vi "模拟量输入自动测试一组_fast_OK.vi"(8 "AD选择？":bool, 9 "DSP选择？":bool, 11 "第几个":i32) -> ()   [LabVIEW 2010]
uses:
  全局量/试验配置信息.vi
panel:
  in  "AD测试值":dbl[](array[numeric])
  in  "DSP测试值":dbl[](array[numeric])
  # "从0开始"
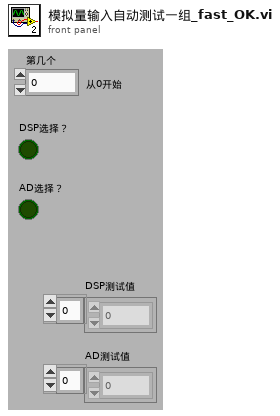
[diagram p1: front panel]
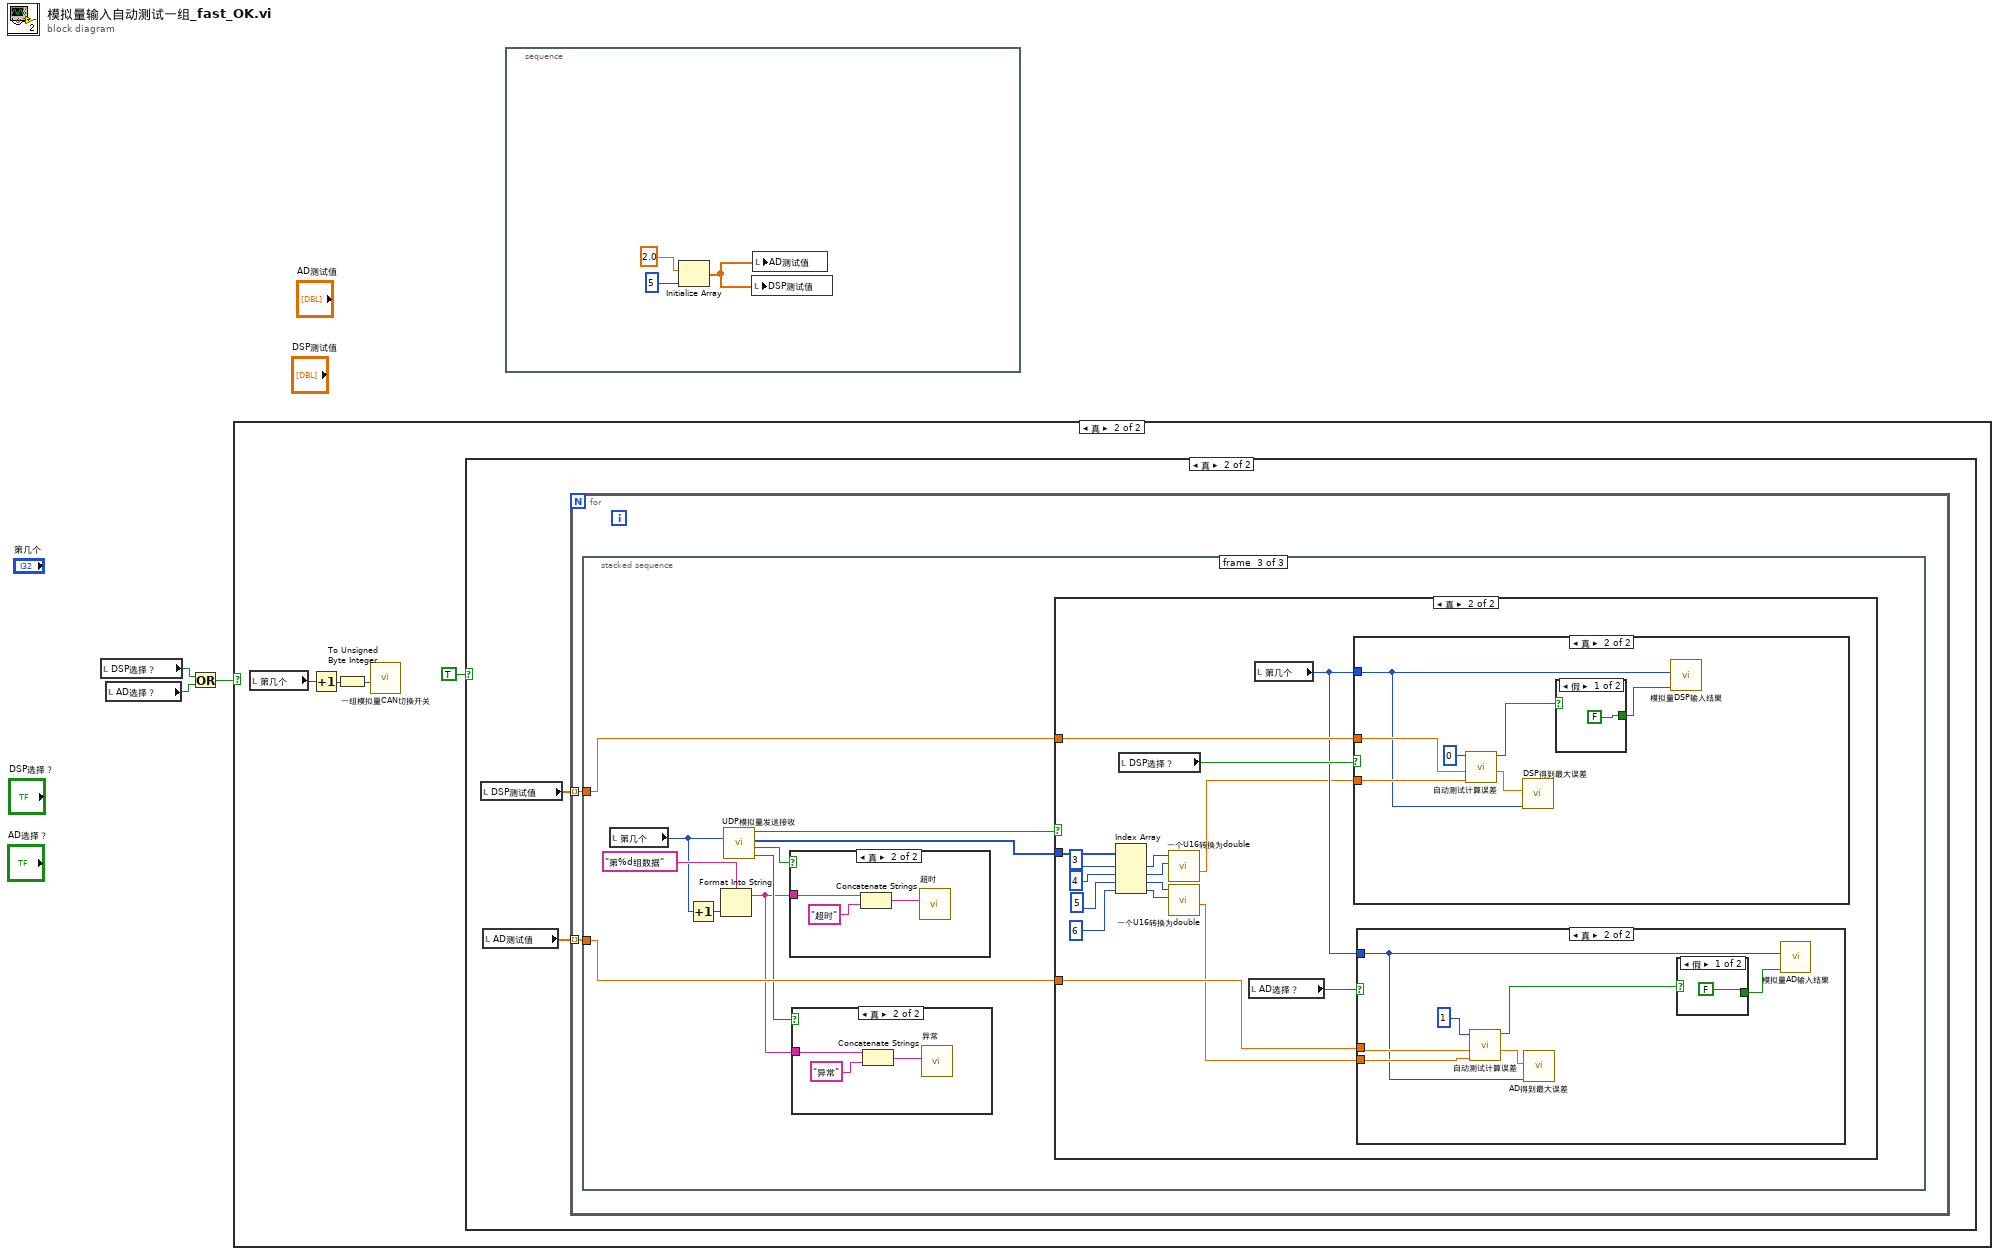
[diagram p0: block diagram]
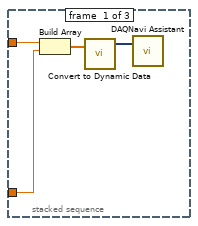
[diagram p4: hidden frame]
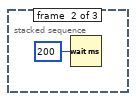
[diagram p5: hidden frame]
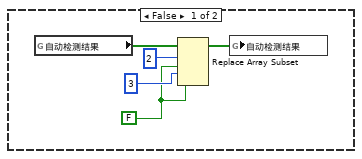
[diagram p8: hidden frame]
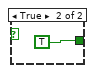
[diagram p10: hidden frame]
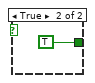
[diagram p12: hidden frame]
diagram:
  n1 = local read "DSP选择？"() -> (w2:bool)
  n2 = local read "AD选择？"() -> (w3:bool)
  n3 = Or(x=w2, y=w3) -> (x .or. y?=w1:bool)
  n4 = case shown="真" w1 {
    frame False {
    }
    frame True {
      n5 = local read "第几个"() -> (w7:i32)
      n6 = Increment(x=w7) -> (x+1=w5:i32)
      n7 = To Unsigned Byte Integer(number=w5) -> (unsigned 8bit integer=w6:u8)
      n8 = call "一组模拟量CAN切换开关.vi"("第几组数据"=w6) -> ()  [unwired: 10 in, 1 out]
      n9 = case shown="真" TRUE {
        frame False {
        }
        frame True {
          n10 = local read "DSP测试值"() -> (w9:dbl[])
          n11 = local read "AD测试值"() -> (w8:dbl[])
          n12 = for {
            tunnel: w9 -> [w11] mode=indexing
            tunnel: w8 -> [w10] mode=indexing
            n13 = stacked-sequence {
              tunnel: w11 -> [w13 _ w26]
              tunnel: w10 -> [w12 _ w25]
              frame #0 {
                n14 = Build Array(w13, w12) -> (w15:dbl[])
                n15 = call "Convert to Dynamic Data"("Array"=w15) -> ("Dynamic Data Type"=w14:dynamicdata)  [unwired: 3 out]
                n16 = call "DAQNavi Assistant"("data in(DDT)"=w14) -> ()  [unwired: 2 in, 17 out]
              }
              frame #1 {
                n17 = Wait (ms)(milliseconds to wait=u32 200 ("等待时间（毫秒）")) -> ()  [unwired: 1 out]
              }
              frame #2 {
                n18 = local read "第几个"() -> (w18:i32)
                n19 = Increment(x=w18) -> (x+1=w19:i32)
                n20 = Format Into String(format string="第%d组数据" ("格式字符串"), w19) -> (resulting string=w20:string)  [unwired: 2 in, 1 out]
                n21 = call "UDP模拟量发送接收.vi"("第几组"=w18) -> ("异常_找到?"=w21:bool, "接收超时?"=w17:bool, "接收的一帧数据"=w24:u16[], "正常_找到?"=w23:bool)  [unwired: 7 in]
                n22 = case shown="真" w17 {
                  tunnel: w20 -> [_ w32]
                  frame False {
                  }
                  frame True {
                    n23 = Concatenate Strings(w32, "超时" ("格式字符串")) -> (w30:string)
                    n24 = call "超时"("Message"=w30) -> ()  [unwired: 9 in, 2 out]
                  }
                }
                n25 = case shown="真" w21 {
                  tunnel: w20 -> [_ w29]
                  frame False {
                  }
                  frame True {
                    n26 = Concatenate Strings(w29, "异常" ("格式字符串")) -> (w27:string)
                    n27 = call "异常"("Message"=w27) -> ()  [unwired: 9 in, 2 out]
                  }
                }
                n28 = case shown="真" w23 {
                  tunnel: w24 -> [_ w45]
                  tunnel: w26 -> [_ w43]
                  tunnel: w25 -> [_ w42]
                  frame False {
                    w33 = FALSE
                    n29 = global read "试验配置信息.vi" "自动检测结果"() -> (w36:bool[])
                    n30 = Replace Array Subset(array=w36, new element #1=w33, index #1=2 ("索引"), new element #2=w33, index #2=3 ("索引")) -> (w35:bool[])
                    n31 = global write "试验配置信息.vi" "自动检测结果"(w35) -> ()
                  }
                  frame True {
                    n32 = Index Array(array=w45, index #1=3 ("索引"), index #2=4 ("索引"), index #3=5 ("索引"), index #4=6 ("索引")) -> (element #1=w50:u16, element #2=w51:u16, element #3=w52:u16, element #4=w53:u16)
                    n33 = local read "DSP选择？"() -> (w44:bool)
                    n34 = call "一个U16转换为double.vi"("低16位_1"=w51, "高16位_1"=w50) -> ("反馈值"=w38:dbl)  [unwired: 9 in]
                    n35 = call "一个U16转换为double.vi"("低16位_1"=w53, "高16位_1"=w52) -> ("反馈值"=w41:dbl)  [unwired: 9 in]
                    n36 = local read "AD选择？"() -> (w40:bool)
                    n37 = local read "第几个"() -> (w39:i32)
                    n38 = case shown="真" w44 {
                      tunnel: w43 -> [_ w68]
                      tunnel: w38 -> [_ w67]
                      tunnel: w39 -> [_ w63]
                      frame False {
                      }
                      frame True {
                        n39 = call "自动测试计算误差.vi"("反馈值"=w67, "输入值"=w68, "DSP_OR_AD"=0) -> ("误差"=w64:dbl, "合格？"=w66:bool)  [unwired: 7 in]
                        n40 = call "DSP得到最大误差.vi"("第几组"=w63, "新误差值"=w64) -> ()  [unwired: 10 in]
                        n41 = case shown="假" w66 {
                          tunnel: [FALSE TRUE] -> w65
                          frame False {
                          }
                          frame True {
                          }
                        }
                        n42 = call "模拟量DSP输入结果.vi"("合格?"=w65, "第几个"=w63) -> ()  [unwired: 10 in]
                      }
                    }
                    n43 = case shown="真" w40 {
                      tunnel: w42 -> [_ w58]
                      tunnel: w41 -> [_ w57]
                      tunnel: w39 -> [_ w54]
                      frame False {
                      }
                      frame True {
                        n44 = call "自动测试计算误差.vi"("反馈值"=w57, "输入值"=w58, "DSP_OR_AD"=1) -> ("误差"=w55:dbl, "合格？"=w59:bool)  [unwired: 7 in]
                        n45 = call "AD得到最大误差.vi"("第几组"=w54, "新误差值"=w55) -> ()  [unwired: 10 in]
                        n46 = case shown="假" w59 {
                          tunnel: [FALSE TRUE] -> w56
                          frame False {
                          }
                          frame True {
                          }
                        }
                        n47 = call "模拟量AD输入结果.vi"("合格?"=w56, "第几个"=w54) -> ()  [unwired: 10 in]
                      }
                    }
                  }
                }
              }
            }
          }
        }
      }
    }
  }
  n48 = stacked-sequence {
    frame #0 {
      n49 = Initialize Array(2.0, 5 ("维数大小")) -> (w72:dbl[])
      n50 = local write "DSP测试值"(w72) -> ()
      n51 = local write "AD测试值"(w72) -> ()
    }
  }
